vi "Digital_Bridge_3_kart.vi"() -> ()   [LabVIEW 2014] (continued)
                      }
                    }
                    n2285 = case shown="True" w5611 {
                      frame False {
                      }
                      frame True {
                        n2286 = local write "KONTROL Y 3"(TRUE ("KONTROL Y 4")) -> ()
                      }
                    }
                  }
                  frame #1 {
                    n2287 = local write "RANGE KONTROL X 3"(FALSE ("KONTROL Y 4")) -> ()
                    n2288 = local read "İterasyon X 3"() -> (w5615:dbl)
                    n2289 = Increment(x=w5615) -> (x+1=w5616:dbl)
                    n2290 = local write "İterasyon X 3"(w5616) -> ()
                  }
                }
              }
            }
            n2291 = case shown="True" "RANGE KONTROL Y 3" {
              frame False {
              }
              frame True {
                n2292 = local read "Outpu Denge Kosulu y1_y2"() -> (w5524:dbl[][])
                n2293 = local read "frekans index"() -> (w5517:dbl)
                n2294 = local read "input 1 y [1R]"() -> (w5525:dbl)
                n2295 = local read "iterasyon 1R"() -> (w5523:dbl)
                n2296 = local read "input 2 y [1R]"() -> (w5526:dbl)
                n2297 = local read "output 2 y [1R]"() -> (w5520:dbl)
                n2298 = local read "output 1 y [1R]"() -> (w5522:dbl)
                n2299 = call "Range Kontrol Y.vi"("denge degeri"=3.0, "iterasyon Denge"=w5523, "frekans index"=w5517, "Denge Kosulu y1_y2"=w5524, "Yk"=w5525, "Y(k-1)"=w5526, "output y 1"=w5522, "output y 2"=w5520) -> ("Output Y(k-1)"=w5516:dbl, "result output y"=w5527:dbl, "KONTROL X"=w5519:bool, "IF ELSE"=w5518:bool)  [unwired: 8 in]
                n2300 = local write "1R Y(k-1)"(w5516) -> ()
                n2301 = local write "result output y [1R]"(w5527) -> ()
                n2302 = flat-sequence {
                  tunnel: w5519 -> [w5529]
                  tunnel: w5518 -> [w5528]
                  frame #0 {
                    n2303 = case shown="True" w5528 {
                      frame False {
                      }
                      frame True {
                        n2304 = local write "IF ELSE Y 3"(TRUE ("IF ELSE X 4")) -> ()
                      }
                    }
                    n2305 = case shown="True" w5529 {
                      frame False {
                      }
                      frame True {
                        n2306 = local write "KONTROL X 3"(TRUE ("KONTROL Y 4")) -> ()
                      }
                    }
                  }
                  frame #1 {
                    n2307 = local write "RANGE KONTROL Y 3"(FALSE ("KONTROL Y 4")) -> ()
                    n2308 = local read "İterasyon Y 3"() -> (w5533:dbl)
                    n2309 = Increment(x=w5533) -> (x+1=w5532:dbl)
                    n2310 = local write "İterasyon Y 3"(w5532) -> ()
                  }
                }
              }
            }
            n2311 = case shown="True" "X 3" {
              frame False {
              }
              frame True {
                n2312 = local read "İterasyon X 3"() -> (w5639:dbl)
                n2313 = local read "1R X(k-1)"() -> (w5640:dbl)
                n2314 = call "X.vi"("X(k-1)"=w5640, "İterasyon Denge"=w5639, "denge degeri"=3.0) -> ("error"=w5637:bool, "output X(k-1)"=w5634:dbl, "output x 1"=w5635:dbl, "cycle"=w5636:bool)  [unwired: 5 in]
                n2315 = case shown="False" w5636 {
                  tunnel: w5637 -> [w5643 _]
                  tunnel: w5635 -> [w5642 _]
                  tunnel: w5634 -> [w5641 _]
                  frame False {
                    n2316 = case shown="False" w5643 {
                      frame False {
                        n2317 = local write "X1 3"(TRUE ("X1 4")) -> ()
                        n2318 = local write "X 3"(FALSE ("X 4")) -> ()
                      }
                      frame True {
                        n2319 = local write "error"(TRUE ("error")) -> ()
                        n2320 = local write "X 3"(FALSE ("X 4")) -> ()
                      }
                    }
                    n2321 = local write "1R X(k-1)"(w5641) -> ()
                    n2322 = local write "output 1 x [1R]"(w5642) -> ()
                    n2323 = local write "input 2 x [1R]"(w5641) -> ()
                  }
                  frame True {
                  }
                }
              }
            }
            n2324 = case shown="True" "read x1 y1 3" {
              frame False {
              }
              frame True {
                n2325 = local read "X Range 1R"() -> (w5400:dbl)
                n2326 = call "only_x_and_y_output.vi"("range"=w5400) -> ("cycle 2"=w5404:bool, "range 2"=w5401:dbl, "Output Y"=w5402:dbl, "Output X"=w5403:dbl)  [unwired: 7 in]
                n2327 = case shown="False" w5404 {
                  tunnel: w5403 -> [w5407 _]
                  tunnel: w5402 -> [w5406 _]
                  tunnel: w5401 -> [w5405 w5415]
                  frame False {
                    n2328 = flat-sequence {
                      tunnel: w5407 -> [w5410]
                      tunnel: w5406 -> [w5409]
                      tunnel: w5405 -> [w5408]
                      frame #0 {
                        n2329 = local write "Output Y1"(w5409) -> ()
                        n2330 = local write "X Range 1R"(w5408) -> ()
                        n2331 = local write "Output X1"(w5410) -> ()
                      }
                      frame #1 {
                        n2332 = local read "X 2.input 1R"() -> (w5411:dbl)
                        n2333 = global write "DB_Global_4_kart-Test.vi" "amplitude 3/1"(w5411) -> ()
                      }
                      frame #2 {
                        n2334 = Wait (ms)(milliseconds to wait=u32 750) -> ()  [unwired: 1 out]
                      }
                      frame #3 {
                        n2335 = local write "read x1 y1 3"(FALSE ("output x")) -> ()
                        n2336 = local write "read x2 y2 3"(TRUE ("output x")) -> ()
                      }
                    }
                  }
                  frame True {
                    n2337 = local write "X Range 1R"(w5415) -> ()
                  }
                }
              }
            }
            n2338 = case shown="True" "Y 3" {
              frame False {
              }
              frame True {
                n2339 = local read "İterasyon Y 3"() -> (w5556:dbl)
                n2340 = local read "1R Y(k-1)"() -> (w5557:dbl)
                n2341 = call "Y.vi"("Y(k-1)"=w5557, "İterasyon Denge"=w5556, "denge degeri"=3.0) -> ("error"=w5554:bool, "output Y(k-1)"=w5551:dbl, "output y 1"=w5552:dbl, "cycle"=w5553:bool)  [unwired: 5 in]
                n2342 = case shown="False" w5553 {
                  tunnel: w5554 -> [w5560 _]
                  tunnel: w5552 -> [w5559 _]
                  tunnel: w5551 -> [w5558 _]
                  frame False {
                    n2343 = case shown="False" w5560 {
                      frame False {
                        n2344 = local write "Y1 3"(TRUE ("X1 4")) -> ()
                        n2345 = local write "Y 3"(FALSE ("X 4")) -> ()
                      }
                      frame True {
                        n2346 = local write "error"(TRUE ("error")) -> ()
                        n2347 = local write "Y 3"(FALSE ("X 4")) -> ()
                      }
                    }
                    n2348 = local write "1R Y(k-1)"(w5558) -> ()
                    n2349 = local write "input 2 y [1R]"(w5558) -> ()
                    n2350 = local write "output 1 y [1R]"(w5559) -> ()
                  }
                  frame True {
                  }
                }
              }
            }
            n2351 = case shown="True" "Y1 3" {
              frame False {
              }
              frame True {
                n2352 = local read "İterasyon Y 3"() -> (w5540:dbl)
                n2353 = local read "output 1 y [1R]"() -> (w5543:dbl)
                n2354 = local read "1R Y(k-1)"() -> (w5542:dbl)
                n2355 = local read "1R Yk"() -> (w5541:dbl)
                n2356 = call "Y1.vi"("denge degeri"=3.0, "İterasyon Denge"=w5540, "Yk"=w5541, "Y(k-1)"=w5542, "output y 1"=w5543) -> ("Output Yk"=w5536:dbl, "output y 2"=w5535:dbl, "cycle"=w5537:bool, "error"=w5538:bool)  [unwired: 7 in]
                n2357 = case shown="False" w5537 {
                  tunnel: w5538 -> [w5546 _]
                  tunnel: w5536 -> [w5545 _]
                  tunnel: w5535 -> [w5544 _]
                  frame False {
                    n2358 = case shown="False" w5546 {
                      frame False {
                        n2359 = local write "RANGE KONTROL Y 3"(TRUE ("RANGE KONTROL X 4")) -> ()
                        n2360 = local write "Y1 3"(FALSE ("X1 4")) -> ()
                      }
                      frame True {
                        n2361 = local write "Y1 3"(FALSE ("X1 4")) -> ()
                        n2362 = local write "error"(TRUE ("error")) -> ()
                      }
                    }
                    n2363 = local write "1R Yk"(w5545) -> ()
                    n2364 = local write "output 2 y [1R]"(w5544) -> ()
                  }
                  frame True {
                  }
                }
              }
            }
            n2365 = case shown="True" "X1 3" {
              frame False {
              }
              frame True {
                n2366 = local read "İterasyon X 3"() -> (w5623:dbl)
                n2367 = local read "output 1 x [1R]"() -> (w5626:dbl)
                n2368 = local read "1R X(k-1)"() -> (w5625:dbl)
                n2369 = local read "1R Xk"() -> (w5624:dbl)
                n2370 = call "X1.vi"("denge degeri"=3.0, "İterasyon Denge"=w5623, "Xk"=w5624, "X(k-1)"=w5625, "output x 1"=w5626) -> ("Output Xk"=w5619:dbl, "output x 2"=w5618:dbl, "cycle"=w5620:bool, "error"=w5621:bool)  [unwired: 7 in]
                n2371 = case shown="False" w5620 {
                  tunnel: w5621 -> [w5629 _]
                  tunnel: w5619 -> [w5628 _]
                  tunnel: w5618 -> [w5627 _]
                  frame False {
                    n2372 = case shown="True" w5629 {
                      frame False {
                        n2373 = local write "RANGE KONTROL X 3"(TRUE ("RANGE KONTROL X 4")) -> ()
                        n2374 = local write "X1 3"(FALSE ("X1 4")) -> ()
                      }
                      frame True {
                        n2375 = local write "error"(TRUE ("error")) -> ()
                        n2376 = local write "X1 3"(FALSE ("X1 4")) -> ()
                      }
                    }
                    n2377 = local write "1R Xk"(w5628) -> ()
                    n2378 = local write "output 2 x [1R]"(w5627) -> ()
                  }
                  frame True {
                  }
                }
              }
            }
            n2379 = case shown="True" "read x2 y2 3" {
              frame False {
              }
              frame True {
                n2380 = local read "X Range 1R"() -> (w5384:dbl)
                n2381 = call "only_x_and_y_output.vi"("range"=w5384) -> ("cycle 2"=w5388:bool, "range 2"=w5385:dbl, "Output Y"=w5386:dbl, "Output X"=w5387:dbl)  [unwired: 7 in]
                n2382 = case shown="False" w5388 {
                  tunnel: w5387 -> [w5391 _]
                  tunnel: w5386 -> [w5390 _]
                  tunnel: w5385 -> [w5389 w5399]
                  frame False {
                    n2383 = flat-sequence {
                      tunnel: w5391 -> [w5394]
                      tunnel: w5390 -> [w5393]
                      tunnel: w5389 -> [w5392]
                      frame #0 {
                        n2384 = local write "Output X2"(w5394) -> ()
                        n2385 = local write "Output Y2"(w5393) -> ()
                        n2386 = local write "X Range 1R"(w5392) -> ()
                      }
                      frame #1 {
                        n2387 = global write "DB_Global_4_kart-Test.vi" "amplitude 3/1"(0.0) -> ()
                      }
                      frame #2 {
                        n2388 = Wait (ms)(milliseconds to wait=u32 750) -> ()  [unwired: 1 out]
                      }
                      frame #3 {
                        n2389 = local write "result phase 3"(TRUE ("result phase 4")) -> ()
                        n2390 = local write "read x2 y2 3"(FALSE ("output y")) -> ()
                      }
                    }
                  }
                  frame True {
                    n2391 = local write "X Range 1R"(w5399) -> ()
                  }
                }
              }
            }
            n2392 = case shown="True" "IF ELSE X 3" {
              frame False {
              }
              frame True {
                n2393 = local read "input 1 x [1R]"() -> (w5585:dbl)
                n2394 = local read "input 2 x [1R]"() -> (w5586:dbl)
                n2395 = local read "output 1 x [1R]"() -> (w5589:dbl)
                n2396 = local read "result output x [1R]"() -> (w5591:dbl)
                n2397 = local read "output 2 x [1R]"() -> (w5590:dbl)
                n2398 = call "If Else X.vi"("denge degeri"=3.0, "Xk"=w5585, "X(k-1)"=w5586, "output x 1"=w5589, "output x 2"=w5590, "result output x"=w5591) -> ("Output X(k-1)"=w5584:dbl, "Start X"=w5587:bool)  [unwired: 8 in]
                n2399 = local write "1R X(k-1)"(w5584) -> ()
                n2400 = case shown="True" w5587 {
                  frame False {
                  }
                  frame True {
                    n2401 = local read "count meas"() -> (w5592:u16)
                    n2402 = local write "RESET SENS X 3"(TRUE ("START X 4")) -> ()
                    n2403 = local write "IF ELSE X 3"(FALSE ("IF ELSE X 4")) -> ()
                    n2404 = Increment(x=w5592) -> (x+1=w5593:u16)
                    n2405 = local write "count meas"(w5593) -> ()
                  }
                }
              }
            }
            n2406 = case shown="True" "IF ELSE Y 3" {
              frame False {
              }
              frame True {
                n2407 = local read "input 1 y [1R]"() -> (w5505:dbl)
                n2408 = local read "input 2 y [1R]"() -> (w5506:dbl)
                n2409 = local read "output 1 y [1R]"() -> (w5509:dbl)
                n2410 = local read "result output y [1R]"() -> (w5511:dbl)
                n2411 = local read "output 2 y [1R]"() -> (w5510:dbl)
                n2412 = call "If Else Y.vi"("denge degeri"=3.0, "Yk"=w5505, "Y(k-1)"=w5506, "output y 1"=w5509, "output y 2"=w5510, "result output y"=w5511) -> ("Output Y(k-1)"=w5504:dbl, "Start Y"=w5507:bool)  [unwired: 8 in]
                n2413 = local write "1R Y(k-1)"(w5504) -> ()
                n2414 = case shown="True" w5507 {
                  frame False {
                  }
                  frame True {
                    n2415 = local read "count meas"() -> (w5512:u16)
                    n2416 = local write "RESET SENS Y 3"(TRUE ("START X 4")) -> ()
                    n2417 = Increment(x=w5512) -> (x+1=w5513:u16)
                    n2418 = local write "count meas"(w5513) -> ()
                    n2419 = local write "IF ELSE Y 3"(FALSE ("IF ELSE X 4")) -> ()
                  }
                }
              }
            }
            n2420 = case shown="True" "result phase 3" {
              frame False {
              }
              frame True {
                n2421 = flat-sequence {
                  tunnel: [w5425] -> w5424
                  tunnel: w5424 -> [w5445]
                  tunnel: [w5445] -> w5423
                  tunnel: w5423 -> [w5450]
                  tunnel: [w5450] -> w5422
                  tunnel: w5422 -> [w5456]
                  frame #0 {
                    # "pi"
                    n2422 = local read "Output X1"() -> (w5430:dbl)
                    n2423 = local read "Output X2"() -> (w5431:dbl)
                    n2424 = local read "Output Y1"() -> (w5432:dbl)
                    n2425 = local read "Output Y2"() -> (w5433:dbl)
                    n2426 = local read "GPIB In"() -> (w5434:refnum<visa-resource-name>)
                    n2427 = call "return phase.vi"("VISA resource name"=w5434) -> ("return phase"=w5426:string)  [unwired: 10 in]
                    n2428 = Fract/Exp String To Number(use system decimal point (T)=FALSE, string=w5426) -> (number=w5428:dbl)  [unwired: 2 in, 1 out]
                    n2429 = formula code="theta = atan((y2-y1)/(x2-x1))*(180/pi)+phase;"("x1"=w5430, "x2"=w5431, "y1"=w5432, "y2"=w5433, "phase"=w5428, "pi"=3.141592653589793) -> ("theta"=w5425:dbl)
                  }
                  frame #1 {
                    n2430 = local read "frekans index"() -> (w5442:dbl)
                    n2431 = local read "Frekanslar"() -> (w5443:dbl[])
                    n2432 = local read "Cluster 2"() -> (w5437:T1)
                    n2433 = local read "Direnc 1 - Direnc 2"() -> (w5447:u32)
                    n2434 = property on="Default Values Listbox" class="LstBox (strict)"() -> ("Item Names"=w5444:string[])  [unwired: 2 in, 2 out]
                    n2435 = Fract/Exp String To Number(string=w5444) -> (number=w5441:dbl[])  [unwired: 3 in, 1 out]
                    n2436 = Index Array(array=w5443, index=w5442) -> (element=w5439:dbl)
                    n2437 = local read "1R F/P Array"() -> (w5448:dbl[][])
                    n2438 = Search 1D Array(1D array=w5441, element=w5439, start index (0)=0) -> (index of element=w5438:i32)
                    n2439 = Increment(x=w5447) -> (x+1=w5446:u32)
                    n2440 = Replace Array Subset(array=w5448, new element=w5445, index (row)=w5446, index (col)=w5438) -> (w5435:dbl[][])
                    n2441 = Bundle By Name(cluster=w5437, "1R F/P Array"=w5435) -> (w5436:T1)
                    n2442 = local write "1R F/P Array"(w5435) -> ()
                    n2443 = local write "Cluster 2"(w5436) -> ()
                  }
                  frame #2 {
                    n2444 = Wait (ms)(milliseconds to wait=u32 250) -> ()  [unwired: 1 out]
                  }
                  frame #3 {
                    w5453 = u16 0 items=["A", "A-B"] ("Input Source (0: A)")
                    n2445 = local read "GPIB In"() -> (w5452:refnum<visa-resource-name>)
                    n2446 = Number To Fractional String(number=w5456) -> (F-format string=w5457:string)  [unwired: 3 in]
                    n2447 = Search and Replace String(input string=w5457, search string=",", replace string="." ("replace string (\"\")")) -> (result string=w5451:string)  [unwired: 5 in, 3 out]
                    n2448 = call "reference phase.vi"("Reference Phase (0.000 degrees)"=w5451, "VISA resource name"=w5452) -> ("error out"=w5454:errorcluster, "VISA resource name out"=w5455:refnum<visa-resource-name>)  [unwired: 8 in]
                    n2449 = call "input source.vi"("error in (no error)"=w5454, "Input Source (0: A)"=w5453, "VISA resource name"=w5455) -> ()  [unwired: 7 in, 2 out]
                  }
                  frame #4 {
                    n2450 = local write "Contiune 1R"(TRUE ("Contiune Wagner")) -> ()
                    n2451 = local write "result phase 3"(FALSE ("result phase 4")) -> ()
                  }
                }
              }
            }
            n2452 = case shown="True" "KONTROL X 3" {
              frame False {
              }
              frame True {
                n2453 = local read "Output Denge Kosulu x1_x2"() -> (w5493:dbl[][])
                n2454 = local read "iterasyon 1R"() -> (w5485:dbl)
                n2455 = local read "Manuel/Otomatik"() -> (w5492:enum16{"Manuel", "Otomatik"})
                n2456 = local read "frekans index"() -> (w5486:dbl)
                n2457 = call "Kontrol X.vi"("denge degeri"=3.0, "İterasyon Denge"=w5485, "Denge Kosulu x1_x2"=w5493, "Manuel/Otomatik"=w5492, "frekans index"=w5486) -> ("Denge Seçimi"=w5489:u8, "New İterasyon Denge"=w5488:dbl, "Iterasyon Count Successful"=w5487:dbl, "Start Denge X"=w5490:bool)  [unwired: 7 in]
                n2458 = case shown="True" w5490 {
                  tunnel: w5489 -> [_ _]
                  tunnel: w5488 -> [_ _]
                  tunnel: w5487 -> [w5501 _]
                  frame False {
                    n2459 = local write "Iterasyon Successful"(w5501) -> ()
                    n2460 = local write "10R switch"(TRUE ("10R switch")) -> ()
                    n2461 = local read "iterasyon 1R"() -> (w5495:dbl)
                    n2462 = local write "Denge Seçimi"(u8 2 ("Denge Seçimi")) -> ()
                    n2463 = local write "KONTROL X 3"(FALSE ("KONTROL X 3")) -> ()
                    n2464 = local write "count meas"(u16 0 ("count meas")) -> ()
                    n2465 = local write "Boolean 3"(TRUE ("Boolean 4")) -> ()
                    n2466 = Increment(x=w5495) -> (x+1=w5494:dbl)
                    n2467 = local write "iterasyon 1R"(w5494) -> ()
                  }
                  frame True {
                    n2468 = local write "KONTROL X 3"(FALSE ("KONTROL X 3")) -> ()
                    n2469 = local write "RESET SENS X 3"(TRUE ("Start Wagner Y")) -> ()
                  }
                }
              }
            }
            n2470 = case shown="True" "KONTROL Y 3" {
              frame False {
              }
              frame True {
                n2471 = local read "Outpu Denge Kosulu y1_y2"() -> (w5573:dbl[][])
                n2472 = local read "iterasyon 1R"() -> (w5565:dbl)
                n2473 = local read "Manuel/Otomatik"() -> (w5572:enum16{"Manuel", "Otomatik"})
                n2474 = local read "frekans index"() -> (w5566:dbl)
                n2475 = call "Kontrol Y.vi"("denge degeri"=3.0, "İterasyon Denge"=w5565, "Denge Kosulu y1_y2"=w5573, "Manuel/Otomatik"=w5572, "frekans index"=w5566) -> ("Denge Seçimi"=w5569:u8, "New İterasyon Denge"=w5568:dbl, "Iterasyon Count Successful"=w5567:dbl, "Start Denge Y"=w5570:bool)  [unwired: 7 in]
                n2476 = case shown="True" w5570 {
                  tunnel: w5569 -> [_ _]
                  tunnel: w5568 -> [_ _]
                  tunnel: w5567 -> [w5581 _]
                  frame False {
                    n2477 = local write "Iterasyon Successful"(w5581) -> ()
                    n2478 = local write "10R switch"(TRUE ("10R switch")) -> ()
                    n2479 = local read "iterasyon 1R"() -> (w5575:dbl)
                    n2480 = local write "Denge Seçimi"(u8 2 ("Denge Seçimi")) -> ()
                    n2481 = local write "count meas"(u16 0 ("count meas")) -> ()
                    n2482 = local write "KONTROL Y 3"(FALSE ("KONTROL Y 3")) -> ()
                    n2483 = local write "Boolean 3"(TRUE ("Boolean 4")) -> ()
                    n2484 = Increment(x=w5575) -> (x+1=w5574:dbl)
                    n2485 = local write "iterasyon 1R"(w5574) -> ()
                  }
                  frame True {
                    n2486 = local write "KONTROL Y 3"(FALSE ("KONTROL Y 3")) -> ()
                    n2487 = local write "RESET SENS Y 3"(TRUE ("Start Wagner Y")) -> ()
                  }
                }
              }
            }
          }
          frame 4, Default {
            # "Bu bölümde, ilgili denge durumunun dengede olup olmadığı kontrol edilir.\n\nEğer denge sağlanmışsa, program doğrudan bir sonraki denge aşamasına geçer.\n\nAyrıca, tüm dengeler başarıyla tamamlanmış ve belirlenen ölçüm sayısına ulaşılmışsa, veriler bu alt program (subVI) aracılığıyla Excel dosyasına aktarılır."
            # "Bu bölümde, Y değerinin dengelendiği kabul edilerek, şimdi sıra X değerinin dengede olup olmadığını kontrol etmeye gelir. \n\nEğer X de dengedeyse, program bir sonraki işlem için ilgili switch case’i aktif eder. \n\nAncak Y dengede değilse, program X’i dengelemeye yönelik işlemlere yönlendirilir."
            # "Bu bölümde, X değerinin dengelendiği kabul edilerek, şimdi sıra Y değerinin dengede olup olmadığını kontrol etmeye gelir. \n\nEğer Y de dengedeyse, program bir sonraki işlem için ilgili switch case’i aktif eder. \n\nAncak Y dengede değilse, program Y’yi dengelemeye yönelik işlemlere yönlendirilir."
            # "Bu bölümün temel amacı, ölçüm aralığını (range) artırmaktır. Program, cihazdan gelen X ve Y değerlerini okuyarak bu değerlerin belirlenen aralık içinde olup olmadığını kontrol eder. \n\nEğer değerler aralık dışındaysa, aralık tekrar artırılır ve ölçüm yeniden yapılır. \n\nAyrıca, bu süreçte input ve output değerleri global değişkenlere kaydedilir. Çünkü sonraki turda, bu kaydedilen değerler farklı bir ölçüm aralığında eğim hesaplaması için kullanılacaktır."
            # "Bu bölümde, sıfırlanacak değer cihazdan okunur. Eğer okunan değer denge koşulunu sağlıyorsa, program Kontrol Y Case’ine geçer. \n\nAncak denge koşulu sağlanmazsa, program if-else yapısına yönlendirilir ve buna göre işlem devam eder."
            # "Bu bölümde, cihaza ikinci input değeri uygulanır ve karşılık gelen output değeri okunur. Daha sonra, hem input hem de output değerleri bir formüle yerleştirilir. Bu formül sayesinde, cihazın 0’a eşitleyeceği (sıfırlayacağı) yeni bir input değeri hesaplanır ve bu değer cihaza uygulanır."
            # "Bu bölümde ilk olarak giriş (input) değeri sisteme uygulanır. Eğer program ilk kez çalıştırılıyorsa, global input üzerinden belirlenen ilk değer (genellikle 0 V) kullanılır. \n\nArdından, cihazdan X değerleri okunur. Bu işlem 10 kez tekrarlanır ve elde edilen ölçümlerin ortalaması alınarak bir sonuç değeri elde edilir. Bu ortalama değer, daha sonra yapılacak işlemlerde kullanılmak üzere saklanır. Özellikle, formül içinde X değerini sıfırlamak için bu bilgiye ihtiyaç duyulur. \n\nEğer girilen input değeri 8 V’tan büyükse, bu durum sistem için güvenli olmayabileceğinden program hata (error) verir ve işlemi durdurur."
            # "Auto Phase, Read X1 Y1, Read X2 Y2, Result Phase: \n\nBu bölümler genel olarak faz ölçümü işlemini gerçekleştirir. \n\nİlk olarak, faz değeri 0’a sıfırlanır. Ardından, global input üzerinden belirlenen range (ölçüm aralığı) değeri uygulanır. Bu işlemden sonra yine global input’ta tanımlanmış olan: \n\nInput 1 verilir ve okuma yapılır (Read X1 Y1) \n\nInput 2 verilir ve okuma yapılır (Read X2 Y2) \n\nBu iki ölçüm sonucuna göre faz değeri bir formül yardımıyla hesaplanır. Elde edilen bu yeni faz değeri, ilgili F/P (frekans/faz) dizisine aktarılır. \n\nBu işlemler, sistemin doğru fazla çalışmasını sağlamak ve sonraki işlemlerde bu bilgiyi referans olarak kullanmak için gerçekleştirilir."
            # "X1 4 ile benzer görevi üstleniyor sadece değerler Y oluyor"
            # "X 4 ile benzer görevi üstleniyor sadece değerler Y oluyor"
            # "IF ELSE X 4 ile benzer görevi üstleniyor sadece değerler Y oluyor"
            # "Range Kontrol X 4 ile benzer görevi üstleniyor sadece değerler Y oluyor"
            # "Start X 4 ile benzer görevi üstleniyor sadece değerler Y oluyor"
            # "Reset Sens X 4 ile benzer görevi üstleniyor sadece değerler Y oluyor"
            # "Start Wagner X ile benzer görevi üstleniyor sadece değerler Y oluyor"
            # "dummy fix false ise aynı frekans birden fazla kez ölçmesi için değerler ayarlanmıs true ise farklı frekans için ayarlanmış"
            # "Pass subvi girmeden önce doğru range miyiz değil miyiz ölçüyor, değil ise +2 üst kademeye gidiyor,\n[Sadece wagner'e özel fix default kısmı gelebilir çünkü frekans değişimde ilk başta değerler cihazdan tam okunmuyor fix ise bu sorunu düzeltiryor]"
            # "Bu bölümde, ölçüm için gerekli olan giriş (input) değerleri sisteme girilir. Girişler tamamlandıktan sonra program, ölçüm işlemini başlatmak üzere X adlı bölüme yönlendirilir. Bu adım, ölçüm sürecinin fiilen başlatıldığı ilk noktadır."
            # "Bu bölümde öncelikle, sistemin kaç kez ölçüm yaptığına işaret eden meas number (ölçüm sayısı) kontrol edilir. \nEğer bu sayı 6’dan büyükse (bu sınır kullanıcı tarafından belirlenmiştir ve değiştirilebilir), program hata verir ve reset values adlı bölüme yönlenir. Bu durum, sistemin çok fazla başarısız deneme yapmasını engellemek içindir. \nEğer ölçüm sayısı 6’dan küçükse, program global bir değişken olan sensitivity (duyarlılık) değerini ayarlar ve ardından işlemlere devam etmek üzere Start X bölümüne geçer."
            # "Bu bölümde, daha önce iterasyon (tekrarlama) yapılıp yapılmadığına bakılarak, programın hangi yöne devam edeceğine karar verilir. \n\nEğer gerekli ise, range kontrolü (ölçüm aralığının uygunluğu) yapılır veya sensitivity ayarlama (cihazın duyarlılığını belirleme) bölümlerine yönlendirilir. Bu sayede sistem, ölçüm koşullarına en uygun şekilde ayarlanarak doğru ve güvenilir sonuçlar elde edilmesi sağlanır."
            # "Bu bölümde, daha önce belirlenen F/P dizilerindeki (frekans/faz değerleri) faz bilgileri, mevcut frekansa göre uygulanır. Ardından, ilgili denge koşulunun daha önce gerçekleştirilip gerçekleştirilmediği kontrol edilir. \nEğer bu denge daha önce sağlanmamışsa, program uygun faz ayarlamasını yapar. Ancak denge daha önce zaten kurulmuşsa, faz ayarı yapılmadan işleme devam edilir. Bu sayede gereksiz tekrarların önüne geçilmiş olur."
            # "Bu bölüm, iterasyona (tekrarlamalı işleme) bağlı olarak Reserve ayarının maksimumda mı yoksa minimumda mı olacağını belirler. Aynı zamanda, ölçüm sürecinin başlangıcında kullanılacak olan sensitivity  değerleri de bu bölümde ayarlanır. Bu ayarlar, ölçüm sırasında cihazın hassasiyetini ve çalışma aralığını doğru şekilde belirlemek için gereklidir."
            # "Wagner"
            n2488 = case shown="True" "wagner switch" {
              frame False {
              }
              frame True {
                n2489 = flat-sequence {
                  frame #0 {
                    n2490 = local read "iterasyon WAGNER"() -> (w6354:dbl)
                    n2491 = Equal?(x=w6354, y=0.0) -> (x = y?=w6352:bool)
                    n2492 = case shown="True" w6352 {
                      frame False {
                      }
                      frame True {
                        n2493 = local read "1 or 10"() -> (w6355:i32)
                        n2494 = case shown="1" w6355 {
                          frame 0, Default {
                          }
                          frame 1 {
                            n2495 = local write "iterasyon WAGNER"(1.0 ("iterasyon WAGNER")) -> ()
                          }
                        }
                      }
                    }
                  }
                  frame #1 {
                    n2496 = local read "iterasyon WAGNER"() -> (w6358:dbl)
                    n2497 = Greater?(x=w6358, y=0.0) -> (0:w6357:bool)
                    n2498 = case shown="True" w6357 {
                      frame False {
                        n2499 = local read "Reserve Wagner"() -> (w6361:u16)
                        n2500 = case shown="0, Default" w6361 {
                          tunnel: ["0" ("Reserve(MAX-MIN)") "1" ("Reserve(MAX-MIN)") "2" ("Reserve(MAX-MIN)")] -> w6360
                          frame 0, Default {
                          }
                          frame 1 {
                          }
                          frame 2 {
                          }
                        }
                        n2501 = local read "GPIB In"() -> (w6362:refnum<visa-resource-name>)
                        n2502 = call "Reserve.vi"("Reserve(MAX-MIN)"=w6360, "VISA resource name"=w6362) -> ()  [unwired: 8 in, 2 out]
                      }
                      frame True {
                        n2503 = local read "GPIB In"() -> (w6367:refnum<visa-resource-name>)
                        n2504 = call "Reserve.vi"("Reserve(MAX-MIN)"="0", "VISA resource name"=w6367) -> ()  [unwired: 8 in, 2 out]
                      }
                    }
                  }
                  frame #2 {
                    n2505 = Wait (ms)(milliseconds to wait=u32 500) -> ()  [unwired: 1 out]
                  }
                  frame #3 {
                    w6370 = u16 0 items=["Wagner", "Ground"] ("Switch")
                    w6371 = u16 1 items=["Open All", "Ana Denge", "10R", "1R"] ("Ring")
                    n2506 = call "mux1.vi"("Ring"=w6371) -> ("error out"=w6372:errorcluster)  [unwired: 9 in]
                    n2507 = property on="Tab Control" class="TabCtl (strict)"("Value"=T4."Wagner" ("Tab Control")) -> ()  [unwired: 2 in, 2 out]
                    n2508 = call "mux2.vi"("Switch"=w6370, "error in (no error)"=w6372) -> ()  [unwired: 6 in, 1 out]
                  }
                  frame #4 {
                    n2509 = Wait (ms)(milliseconds to wait=u32 1000) -> ()  [unwired: 1 out]
                  }
                  frame #5 {
                    n2510 = local read "1 or 10"() -> (w6377:i32)
                    n2511 = local read "İterasyon X 4"() -> (w6380:dbl)
                    n2512 = Equal?(x=w6377, y=1) -> (x = y?=w6376:bool)
                    n2513 = Greater?(x=w6380, y=0.0) -> (0:w6375:bool)
                    n2514 = Or(x=w6375, y=w6376) -> (x .or. y?=w6374:bool)
                    n2515 = case shown="False" w6374 {
                      frame False {
                        n2516 = local read "X Range W"() -> (w6382:dbl)
                        n2517 = local read "Y Range W"() -> (w6381:dbl)
                        n2518 = global write "show_sensitivity.vi" "show sensitivity (wagner  x)"(w6382) -> ()
                        n2519 = global write "show_sensitivity.vi" "show sensitivity (wagner  y)"(w6381) -> ()
                      }
                      frame True {
                        w6383 = 16.0 ("Max. Hassasiyet")
                        n2520 = global write "show_sensitivity.vi" "show sensitivity (wagner  x)"(w6383) -> ()
                        n2521 = global write "show_sensitivity.vi" "show sensitivity (wagner  y)"(w6383) -> ()
                      }
                    }
                  }
                  frame #6 {
                    n2522 = local write "wagner switch"(FALSE ("wagner switch")) -> ()
                    n2523 = local write "Start Wagner X"(TRUE ("START WAGNER")) -> ()
                  }
                }
              }
            }
            n2524 = case shown="True" "Start Wagner X" {
              frame False {
              }
              frame True {
                n2525 = flat-sequence {
                  frame #0 {
                    w6414 = u16 0 items=["A", "A-B"] ("Input Source (0: A)")
                    n2526 = local read "frekans index"() -> (w6409:dbl)
                    n2527 = local read "Frekanslar"() -> (w6410:dbl[])
                    n2528 = local read "Direnc 1 - Direnc 2"() -> (w6411:u32)
                    n2529 = local read "Wagner F/P Array"() -> (w6412:dbl[][])
                    n2530 = Index Array(array=w6410, index=w6409) -> (element=w6408:dbl)
                    n2531 = call "get_phase_element.vi"("index r"=w6411, "hz"=w6408, "Array"=w6412) -> ("element"=w6404:dbl)  [unwired: 8 in]
                    n2532 = Number To Fractional String(number=w6404) -> (F-format string=w6407:string)  [unwired: 3 in]
                    n2533 = local read "GPIB In"() -> (w6413:refnum<visa-resource-name>)
                    n2534 = Search and Replace String(input string=w6407, search string=",", replace string="." ("replace string (\"\")")) -> (result string=w6403:string)  [unwired: 5 in, 3 out]
                    n2535 = call "reference phase.vi"("Reference Phase (0.000 degrees)"=w6403, "VISA resource name"=w6413) -> ("error out"=w6415:errorcluster, "VISA resource name out"=w6416:refnum<visa-resource-name>)  [unwired: 8 in]
                    n2536 = call "input source.vi"("error in (no error)"=w6415, "Input Source (0: A)"=w6414, "VISA resource name"=w6416) -> ()  [unwired: 7 in, 2 out]
                  }
                  frame #1 {
                    n2537 = local read "İterasyon X 4"() -> (w6427:dbl)
                    n2538 = local read "1 or 10"() -> (w6431:i32)
                    n2539 = local read "frekans index"() -> (w6426:dbl)
                    n2540 = local read "control hz array"() -> (w6422:dbl[][])
                    n2541 = Greater?(x=w6427, y=0.0) -> (0:w6428:bool)
                    n2542 = call "change2d.vi"("reset(default false)"=FALSE, "index (col)"=w6426, "index (row)"=2, "read/write(T/F)"=TRUE, "2D Array"=w6422) -> ("result count"=w6421:dbl)  [unwired: 5 in, 1 out]
                    n2543 = Equal?(x=w6431, y=1) -> (x = y?=w6429:bool)
                    n2544 = local read "set"() -> (w6420:u16)
                    n2545 = Or(x=w6428, y=w6429) -> (x .or. y?=w6418:bool)
                    n2546 = Equal?(x=w6421, y=w6420) -> (x = y?=w6419:bool)
                    n2547 = Or(x=w6418, y=w6419) -> (x .or. y?=w6417:bool)
                    n2548 = case shown="False" w6417 {
                      frame False {
                        n2549 = local write "auto phase wagner"(TRUE ("auto phase 10R")) -> ()
                        n2550 = local write "Start Wagner X"(FALSE ("auto phase 10R")) -> ()
                      }
                      frame True {
                        n2551 = local write "Contiune Wagner"(TRUE) -> ()
                        n2552 = local write "Start Wagner X"(FALSE ("START WAGNER")) -> ()
                      }
                    }
                  }
                }
              }
            }
            n2553 = case shown="True" "RESET SENS X 4" {
              frame False {
              }
              frame True {
                n2554 = local read "count meas"() -> (w6333:u16)
                n2555 = local read "iterasyon WAGNER"() -> (w6330:dbl)
                n2556 = Greater?(x=w6333, y=u16 8) -> (0:w6329:bool)
                n2557 = Greater?(x=w6330, y=5.0) -> (0:w6328:bool)
                n2558 = Or(x=w6329, y=w6328) -> (x .or. y?=w6327:bool)
                n2559 = case shown="True" w6327 {
                  frame False {
                    n2560 = flat-sequence {
                      frame #0 {
                        n2561 = global read "show_sensitivity.vi" "show sensitivity (wagner  x)"() -> (w6334:dbl)
                        n2562 = local read "GPIB In"() -> (w6335:refnum<visa-resource-name>)
                        n2563 = call "get_sensitivity.vi"("input 1"=w6334, "SR850 GPIB In"=w6335) -> ()  [unwired: 8 in, 2 out]
                      }
                      frame #1 {
                        n2564 = Wait (ms)(milliseconds to wait=u32 500) -> ()  [unwired: 1 out]
                      }
                      frame #2 {
                        n2565 = local write "RESET SENS X 4"(FALSE ("RESET SENS X")) -> ()
                        n2566 = local write "START X 4"(TRUE ("START X 4")) -> ()
                      }
                    }
                  }
                  frame True {
                    n2567 = local read "iterasyon WAGNER"() -> (w6341:dbl)
                    n2568 = Greater?(x=w6341, y=5.0) -> (0:w6339:bool)
                    n2569 = case shown="False" w6339 {
                      frame False {
                        n2570 = flat-sequence {
                          frame #0 {
                            n2571 = local write "count meas"(u16 9 ("count meas")) -> ()
                            n2572 = local write "RESET SENS X 4"(FALSE ("Start 10R X")) -> ()
                            n2573 = local write "İterasyon X 4"(0.0 ("İterasyon X 4")) -> ()
                          }
                          frame #1 {
                            n2574 = local write "reset values"(TRUE ("Start 10R X")) -> ()
                            n2575 = local write "error"(TRUE ("Start 10R X")) -> ()
                          }
                        }
                      }
                      frame True {
                        n2576 = flat-sequence {
                          frame #0 {
                            n2577 = local write "count meas"(u16 10 ("count meas")) -> ()
                            n2578 = local write "RESET SENS X 4"(FALSE ("Start 10R X")) -> ()
                            n2579 = local write "İterasyon X 4"(0.0 ("İterasyon X 4")) -> ()
                          }
                          frame #1 {
                            n2580 = local write "reset values"(TRUE ("Start 10R X")) -> ()
                            n2581 = local write "error"(TRUE ("Start 10R X")) -> ()
                          }
                        }
                      }
                    }
                  }
                }
              }
            }
            n2582 = case shown="True" "START X 4" {
              frame False {
              }
              frame True {
                n2583 = flat-sequence {
                  frame #0 {
                    n2584 = local read "Wagner  X(k-1)"() -> (w6443:dbl)
                    n2585 = local read "Wagner Xk"() -> (w6442:dbl)
                    n2586 = local write "input 2 x [wagner]"(w6443) -> ()
                    n2587 = local write "input 1 x [wagner]"(w6442) -> ()
                    n2588 = global write "DB_Global_4_kart-Test.vi" "amplitude 1/1"(w6442) -> ()
                  }
                  frame #1 {
                    n2589 = Wait (ms)(milliseconds to wait=u32 500) -> ()  [unwired: 1 out]
                  }
                  frame #2 {
                    n2590 = local write "START X 4"(FALSE ("START X 4")) -> ()
                    n2591 = local write "X 4"(TRUE ("START X")) -> ()
                  }
                  frame #3 {
                  }
                }
              }
            }
            n2592 = case shown="True" "Start Wagner Y" {
              frame False {
              }
              frame True {
                n2593 = flat-sequence {
                  frame #0 {
                    w6397 = u16 0 items=["A", "A-B"] ("Input Source (0: A)")
                    n2594 = local read "frekans index"() -> (w6391:dbl)
                    n2595 = local read "Frekanslar"() -> (w6392:dbl[])
                    n2596 = local read "Direnc 1 - Direnc 2"() -> (w6394:u32)
                    n2597 = local read "Wagner F/P Array"() -> (w6395:dbl[][])
                    n2598 = Index Array(array=w6392, index=w6391) -> (element=w6393:dbl)
                    n2599 = call "get_phase_element.vi"("index r"=w6394, "hz"=w6393, "Array"=w6395) -> ("element"=w6387:dbl)  [unwired: 8 in]
                    n2600 = Number To Fractional String(number=w6387) -> (F-format string=w6388:string)  [unwired: 3 in]
                    n2601 = local read "GPIB In"() -> (w6396:refnum<visa-resource-name>)
                    n2602 = Search and Replace String(input string=w6388, search string=",", replace string="." ("replace string (\"\")")) -> (result string=w6386:string)  [unwired: 5 in, 3 out]
                    n2603 = call "reference phase.vi"("Reference Phase (0.000 degrees)"=w6386, "VISA resource name"=w6396) -> ("error out"=w6398:errorcluster, "VISA resource name out"=w6399:refnum<visa-resource-name>)  [unwired: 8 in]
                    n2604 = call "input source.vi"("error in (no error)"=w6398, "Input Source (0: A)"=w6397, "VISA resource name"=w6399) -> ()  [unwired: 7 in, 2 out]
                  }
                  frame #1 {
                    n2605 = local write "RESET SENS Y 4"(TRUE ("START X")) -> ()
                    n2606 = local write "Start Wagner Y"(FALSE ("START Y 6")) -> ()
                    n2607 = local write "Boolean 4"(FALSE ("Boolean 4")) -> ()
                  }
                }
              }
            }
            n2608 = case shown="True" "Optimum Range 4" {
              frame False {
              }
              frame True {
                n2609 = flat-sequence {
                  frame #0 {
                    n2610 = global read "show_sensitivity.vi" "show sensitivity (wagner  x)"() -> (w5934:dbl)
                    n2611 = local read "GPIB In"() -> (w5933:refnum<visa-resource-name>)
                    n2612 = call "get_sensitivity.vi"("input 1"=w5934, "SR850 GPIB In"=w5933) -> ()  [unwired: 8 in, 2 out]
                  }
                  frame #1 {
                    n2613 = call "set optimum range.vi"("denge degeri"=4.0) -> ("ok"=w5935:bool)  [unwired: 14 in]
                    n2614 = case shown="True" w5935 {
                      frame False {
                      }
                      frame True {
                        n2615 = local write "Optimum Range 4"(FALSE ("Optimum Range 1")) -> ()
                        n2616 = local write "PASS WAGNER"(TRUE ("PASS WAGNER")) -> ()
                      }
                    }
                  }
                }
              }
            }
            n2617 = case shown="True" "RESET SENS Y 4" {
              frame False {
              }
              frame True {
                n2618 = local read "count meas"() -> (w6307:u16)
                n2619 = local read "iterasyon WAGNER"() -> (w6305:dbl)
                n2620 = Greater?(x=w6307, y=u16 8) -> (0:w6304:bool)
                n2621 = Greater?(x=w6305, y=5.0) -> (0:w6303:bool)
                n2622 = Or(x=w6304, y=w6303) -> (x .or. y?=w6302:bool)
                n2623 = case shown="True" w6302 {
                  frame False {
                    n2624 = flat-sequence {
                      frame #0 {
                        n2625 = global read "show_sensitivity.vi" "show sensitivity (wagner  y)"() -> (w6309:dbl)
                        n2626 = local read "GPIB In"() -> (w6310:refnum<visa-resource-name>)
                        n2627 = call "get_sensitivity.vi"("input 1"=w6309, "SR850 GPIB In"=w6310) -> ()  [unwired: 8 in, 2 out]
                      }
                      frame #1 {
                        n2628 = Wait (ms)(milliseconds to wait=u32 500) -> ()  [unwired: 1 out]
                      }
                      frame #2 {
                        n2629 = local write "RESET SENS Y 4"(FALSE ("RESET SENS X")) -> ()
                        n2630 = local write "START Y 4"(TRUE ("START X 4")) -> ()
                      }
                    }
                  }
                  frame True {
                    n2631 = local read "iterasyon WAGNER"() -> (w6316:dbl)
                    n2632 = Greater?(x=w6316, y=5.0) -> (0:w6314:bool)
                    n2633 = case shown="False" w6314 {
                      frame False {
                        n2634 = flat-sequence {
                          frame #0 {
                            n2635 = local write "İterasyon X 4"(0.0 ("İterasyon X 4")) -> ()
                            n2636 = local write "count meas"(u16 9 ("count meas")) -> ()
                            n2637 = local write "RESET SENS Y 4"(FALSE ("Start 10R X")) -> ()
                          }
                          frame #1 {
                            n2638 = local write "reset values"(TRUE ("Start 10R X")) -> ()
                            n2639 = local write "error"(TRUE ("Start 10R X")) -> ()
                          }
                        }
                      }
                      frame True {
                        n2640 = flat-sequence {
                          frame #0 {
                            n2641 = local write "İterasyon X 4"(0.0 ("İterasyon X 4")) -> ()
                            n2642 = local write "count meas"(u16 10 ("count meas")) -> ()
                            n2643 = local write "RESET SENS Y 4"(FALSE ("Start 10R X")) -> ()
                          }
                          frame #1 {
                            n2644 = local write "reset values"(TRUE ("Start 10R X")) -> ()
                            n2645 = local write "error"(TRUE ("Start 10R X")) -> ()
                          }
                        }
                      }
                    }
                  }
                }
              }
            }
            n2646 = case shown="True" "START Y 4" {
              frame False {
              }
              frame True {
                n2647 = flat-sequence {
                  frame #0 {
                    n2648 = local read "Wagner Y(k-1)"() -> (w6438:dbl)
                    n2649 = local read "Wagner Yk"() -> (w6437:dbl)
                    n2650 = local write "input 2 y [wagner]"(w6438) -> ()
                    n2651 = local write "input 1 y [wagner]"(w6437) -> ()
                    n2652 = global write "DB_Global_4_kart-Test.vi" "phase 1/1"(w6437) -> ()
                  }
                  frame #1 {
                    n2653 = Wait (ms)(milliseconds to wait=u32 500) -> ()  [unwired: 1 out]
                  }
                  frame #2 {
                    n2654 = local write "START Y 4"(FALSE ("START X")) -> ()
                    n2655 = local write "Y 4"(TRUE ("START X")) -> ()
                  }
                }
              }
            }
            n2656 = case shown="True" "fix default" {
              frame False {
              }
              frame True {
                n2657 = local read "dummy fix default"() -> (w6034:bool)
                n2658 = case shown="False" w6034 {
                  frame False {
                    n2659 = local read "frekans index"() -> (w6035:dbl)
                    n2660 = local read "default values"() -> (w6036:T3)
                    n2661 = call "fix default 2.vi"("frekans index"=w6035, "default values"=w6036) -> ("fix default"=w6037:bool)  [unwired: 9 in]
                    n2662 = case shown="True" w6037 {
                      frame False {
                      }
                      frame True {
                        n2663 = flat-sequence {
                          frame #0 {
                            n2664 = local write "dummy fix default"(TRUE ("PASS WAGNER")) -> ()
                            n2665 = local write "Optimum Range 4"(TRUE ("PASS WAGNER")) -> ()
                            n2666 = local write "fix default"(FALSE ("fix default")) -> ()
                          }
                          frame #1 {
                            n2667 = Wait (ms)(milliseconds to wait=u32 500) -> ()  [unwired: 1 out]
                          }
                          frame #2 {
                          }
                        }
                      }
                    }
                  }
                  frame True {
                    n2668 = local read "input values"() -> (w6043:dbl[])
                    n2669 = call "fix default.vi"("input values"=w6043) -> ("fix default"=w6042:bool)  [unwired: 9 in]
                    n2670 = case shown="True" w6042 {
                      frame False {
                      }
                      frame True {
                        n2671 = flat-sequence {
                          frame #0 {
                            n2672 = local write "Optimum Range 4"(TRUE ("PASS WAGNER")) -> ()
                            n2673 = local write "fix default"(FALSE ("fix default")) -> ()
                          }
                          frame #1 {
                            n2674 = Wait (ms)(milliseconds to wait=u32 500) -> ()  [unwired: 1 out]
                          }
                          frame #2 {
                          }
                        }
                      }
                    }
                  }
                }
              }
            }
            n2675 = case shown="True" "Contiune Wagner" {
              frame False {
              }
              frame True {
                n2676 = local read "1 or 10"() -> (w6021:i32)
                n2677 = local read "iterasyon WAGNER"() -> (w6025:dbl)
                n2678 = local read "frekans index"() -> (w6014:dbl)
                n2679 = local read "control hz array"() -> (w6018:dbl[][])
                n2680 = call "change2d.vi"("reset(default false)"=FALSE, "index (col)"=w6014, "index (row)"=2, "read/write(T/F)"=TRUE, "2D Array"=w6018) -> ("result count"=w6019:dbl)  [unwired: 5 in, 1 out]
                n2681 = case shown="1" w6021 {
                  tunnel: [FALSE TRUE] -> w6023
                  frame 10, Default {
                  }
                  frame 1 {
                  }
                }
                n2682 = local read "set"() -> (w6020:u16)
                n2683 = Equal?(x=w6019, y=w6020) -> (x = y?=w6013:bool)
                n2684 = Greater?(x=w6025, y=0.0) -> (0:w6022:bool)
                n2685 = Or(x=w6022, y=w6023) -> (x .or. y?=w6012:bool)
                n2686 = Or(x=w6012, y=w6013) -> (x .or. y?=w6011:bool)
                n2687 = case shown="True" w6011 {
                  frame False {
                    n2688 = local write "Contiune Wagner"(FALSE ("START WAGNER")) -> ()
                    n2689 = local write "RESET SENS X 4"(TRUE ("START X")) -> ()
                    n2690 = local write "Boolean 4"(FALSE ("Boolean 4")) -> ()
                  }
                  frame True {
                    n2691 = local write "Contiune Wagner"(FALSE ("Optimum Range 1")) -> ()
                    n2692 = local write "Boolean 4"(FALSE ("Boolean 4")) -> ()
                    n2693 = local write "fix default"(TRUE ("START X")) -> ()
                  }
                }
              }
            }
            n2694 = case shown="True" "PASS WAGNER" {
              frame False {
              }
              frame True {
                n2695 = flat-sequence {
                  frame #0 {
                  }
                  frame #1 {
                    n2696 = Wait (ms)(milliseconds to wait=u32 500) -> ()  [unwired: 1 out]
                  }
                  frame #2 {
                    n2697 = local read "Other Array"() -> (w6164:dbl[])
                    n2698 = for {
                      N: 7 -> [_]
                      shift-right: [w6198] -> w6167
                      shift-left: w6164 -> [w6201]
                      i -> [w6200]
